vi "FPGA Main v0.vi"() -> ()   [LabVIEW 2017]
uses:
  <vilib>/rvi/Emulation/niFpgaGetClockAttributes.vi
  <vilib>/rvi/Emulation/niFpgaSctlEmulationGetInTimedLoop.vi
  <vilib>/rvi/Emulation/niFpgaEmulationReportErrorSimple.vi
  <vilib>/rvi/eio/common/nirviEmuTemplateMethod_errors.vi
  <vilib>/rvi/Emulation/niFpgaCriticalErrorInLSC.vi
  <vilib>/eio/EIONode/EIONode.xnode
  <vilib>/rvi/FXPMathLib/FxpSub/XNode/nifxpmath_Sub.xnode
  <vilib>/rvi/FXPMathLib/sim/FxpSim.dll
panel:
  in  "DO 1":T1
  out "DI 2":T2
  out "DI 1":T3
  in  "Loop Time (ms)":u32=1 caption="Count(mSec)"
  in  "Stop Button":bool
  out "AI3":fxp<+/-,27,6> format="%.23g"
  out "AI2":fxp<+/-,27,6> format="%.23g"
  out "AI1":fxp<+/-,27,6> format="%.23g"
  out "AI0":fxp<+/-,27,6> format="%.23g"
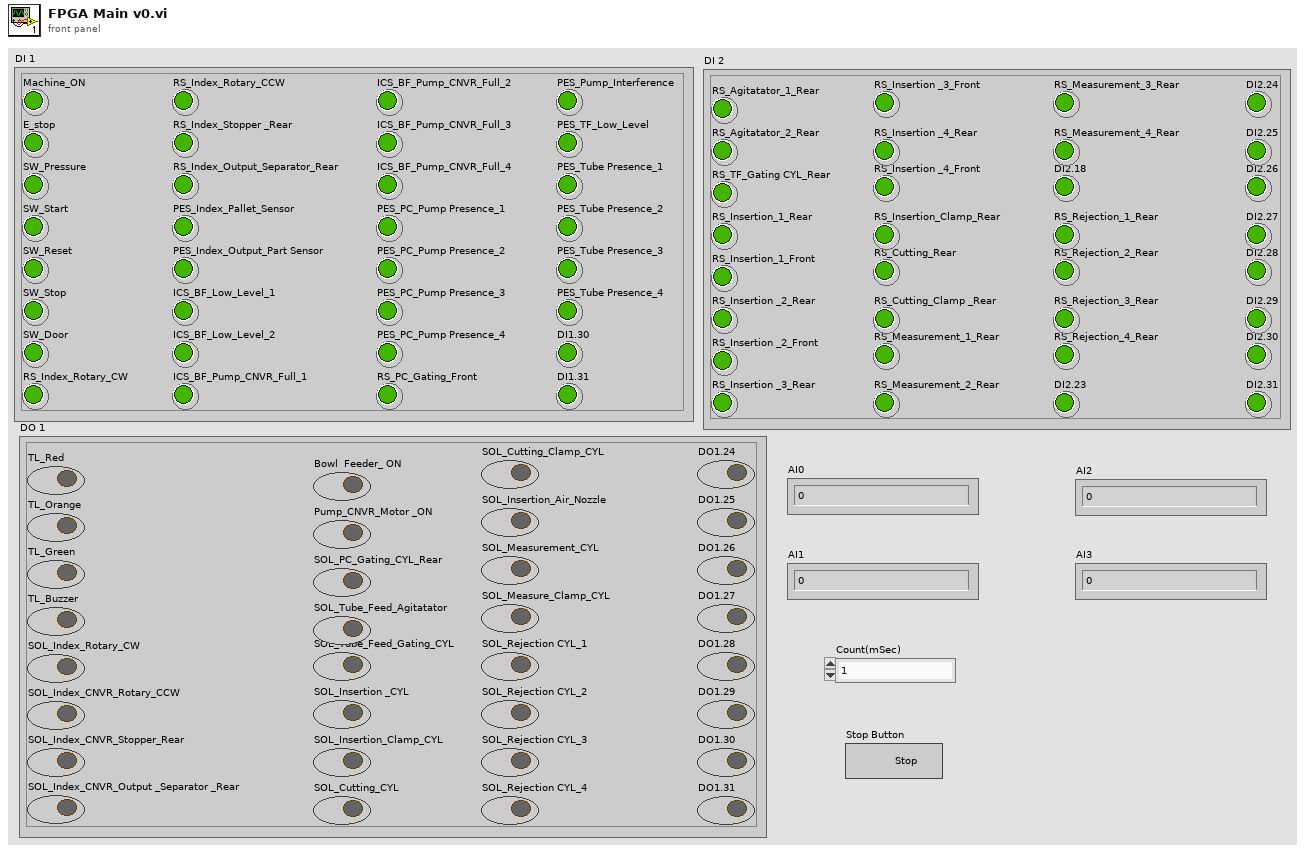
[diagram p1: front panel]
types:
  T1 = cluster{"TL_Red":bool, "TL_Orange":bool, "TL_Green":bool, "TL_Buzzer":bool, "SOL_Index_Rotary_CW":bool, "SOL_Index_CNVR_Rotary_CCW":bool, "SOL_Index_CNVR_Stopper_Rear":bool, "SOL_Index_CNVR_Output _Separator _Rear":bool, "Bowl  Feeder_ ON":bool, "Pump_CNVR_Motor _ON":bool, "SOL_PC_Gating_CYL_Rear":bool, "SOL_Tube_Feed_Agitatator":bool, "SOL_Tube_Feed_Gating_CYL":bool, "SOL_Insertion _CYL":bool, "SOL_Insertion_Clamp_CYL":bool, "SOL_Cutting_CYL":bool, "SOL_Cutting_Clamp_CYL":bool, "SOL_Insertion_Air_Nozzle":bool, "SOL_Measurement_CYL":bool, "SOL_Measure_Clamp_CYL":bool, "SOL_Rejection CYL_1":bool, "SOL_Rejection CYL_2":bool, "SOL_Rejection CYL_3":bool, "SOL_Rejection CYL_4":bool, "DO1.24":bool, "DO1.25":bool, "DO1.26":bool, "DO1.27":bool, "DO1.28":bool, "DO1.29":bool, "DO1.30":bool, "DO1.31":bool}
  T2 = cluster{"RS_Agitatator_1_Rear ":bool, "RS_Agitatator_2_Rear ":bool, "RS_TF_Gating CYL_Rear":bool, "RS_Insertion_1_Rear":bool, "RS_Insertion_1_Front":bool, "RS_Insertion _2_Rear":bool, "RS_Insertion _2_Front":bool, "RS_Insertion _3_Rear":bool, "RS_Insertion _3_Front":bool, "RS_Insertion _4_Rear":bool, "RS_Insertion _4_Front":bool, "RS_Insertion_Clamp_Rear":bool, "RS_Cutting_Rear":bool, "RS_Cutting_Clamp _Rear":bool, "RS_Measurement_1_Rear":bool, "RS_Measurement_2_Rear":bool, "RS_Measurement_3_Rear":bool, "RS_Measurement_4_Rear":bool, "DI2.18":bool, "RS_Rejection_1_Rear":bool, "RS_Rejection_2_Rear":bool, "RS_Rejection_3_Rear":bool, "RS_Rejection_4_Rear":bool, "DI2.23":bool, "DI2.24":bool, "DI2.25":bool, "DI2.26":bool, "DI2.27":bool, "DI2.28":bool, "DI2.29":bool, "DI2.30":bool, "DI2.31":bool}
  T3 = cluster{"Machine_ON":bool, "E_stop ":bool, "SW_Pressure":bool, "SW_Start ":bool, "SW_Reset":bool, "SW_Stop":bool, "SW_Door":bool, "RS_Index_Rotary_CW":bool, "RS_Index_Rotary_CCW":bool, "RS_Index_Stopper _Rear":bool, "RS_Index_Output_Separator_Rear":bool, "PES_Index_Pallet_Sensor":bool, "PES_Index_Output_Part Sensor":bool, "ICS_BF_Low_Level_1":bool, "ICS_BF_Low_Level_2":bool, "ICS_BF_Pump_CNVR_Full_1":bool, "ICS_BF_Pump_CNVR_Full_2":bool, "ICS_BF_Pump_CNVR_Full_3":bool, "ICS_BF_Pump_CNVR_Full_4":bool, "PES_PC_Pump Presence_1":bool, "PES_PC_Pump Presence_2":bool, "PES_PC_Pump Presence_3":bool, "PES_PC_Pump Presence_4":bool, "RS_PC_Gating_Front":bool, "PES_Pump_Interference":bool, "PES_TF_Low_Level":bool, "PES_Tube Presence_1":bool, "PES_Tube Presence_2":bool, "PES_Tube Presence_3":bool, "PES_Tube Presence_4":bool, "DI1.30":bool, "DI1.31":bool}
  T4 = cluster{"Boolean array[0]":bool, "Boolean array[1]":bool, "Boolean array[2]":bool, "Boolean array[3]":bool, "Boolean array[4]":bool, "Boolean array[5]":bool, "Boolean array[6]":bool, "Boolean array[7]":bool, "Boolean array[8]":bool, "Boolean array[9]":bool, "Boolean array[10]":bool, "Boolean array[11]":bool, "Boolean array[12]":bool, "Boolean array[13]":bool, "Boolean array[14]":bool, "Boolean array[15]":bool, "Boolean array[16]":bool, "Boolean array[17]":bool, "Boolean array[18]":bool, "Boolean array[19]":bool, "Boolean array[20]":bool, "Boolean array[21]":bool, "Boolean array[22]":bool, "Boolean array[23]":bool, "Boolean array[24]":bool, "Boolean array[25]":bool, "Boolean array[26]":bool, "Boolean array[27]":bool, "Boolean array[28]":bool, "Boolean array[29]":bool, "Boolean array[30]":bool, "Boolean array[31]":bool}
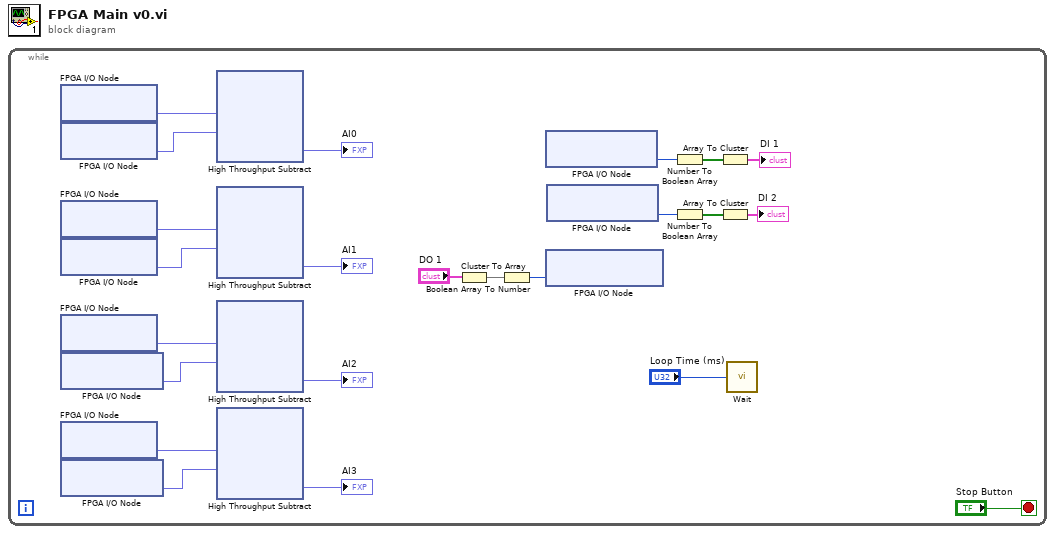
[diagram p0: block diagram]
diagram:
  n1 = while {
    stop <- "Stop Button" stop-if-true
    n2 = xnode "FPGA I/O Node"() -> ("Mod1/AI0"=w23:fxp<+/-,26,5>)  [unwired: 1 in, 1 out]
    n3 = xnode "FPGA I/O Node"() -> ("Mod1/AI8"=w22:fxp<+/-,26,5>)  [unwired: 1 in, 1 out]
    n4 = xnode "FPGA I/O Node"() -> ("Mod1/AI1"=w19:fxp<+/-,26,5>)  [unwired: 1 in, 1 out]
    n5 = xnode "FPGA I/O Node"() -> ("Mod1/AI9"=w18:fxp<+/-,26,5>)  [unwired: 1 in, 1 out]
    n6 = xnode "FPGA I/O Node"() -> ("Mod1/AI2"=w16:fxp<+/-,26,5>)  [unwired: 1 in, 1 out]
    n7 = xnode "FPGA I/O Node"() -> ("Mod1/AI10"=w15:fxp<+/-,26,5>)  [unwired: 1 in, 1 out]
    n8 = xnode "FPGA I/O Node"() -> ("Mod1/AI3"=w13:fxp<+/-,26,5>)  [unwired: 1 in, 1 out]
    n9 = xnode "FPGA I/O Node"() -> ("Mod1/AI11"=w12:fxp<+/-,26,5>)  [unwired: 1 in, 1 out]
    n10 = xnode "High Throughput Subtract"("x"=w23, "y"=w22) -> ("x-y"=→"AI0":fxp<+/-,27,6>)
    n11 = xnode "High Throughput Subtract"("x"=w19, "y"=w18) -> ("x-y"=→"AI1":fxp<+/-,27,6>)
    n12 = xnode "High Throughput Subtract"("x"=w16, "y"=w15) -> ("x-y"=→"AI2":fxp<+/-,27,6>)
    n13 = xnode "High Throughput Subtract"("x"=w13, "y"=w12) -> ("x-y"=→"AI3":fxp<+/-,27,6>)
    n14 = Cluster To Array(cluster="DO 1") -> (array=w3:bool[])
    n15 = Boolean Array To Number(Boolean array=w3) -> (number=w8:u32)
    n16 = xnode "FPGA I/O Node"() -> ("Mod2/DI31:0"=w10:u32)  [unwired: 1 in, 1 out]
    n17 = xnode "FPGA I/O Node"("Mod4/DO31:0"=w8) -> ()  [unwired: 1 in, 1 out]
    n18 = xnode "FPGA I/O Node"() -> ("Mod3/DI31:0"=w9:u32)  [unwired: 1 in, 1 out]
    n19 = Number To Boolean Array(number=w10) -> (Boolean array=w6:bool[])
    n20 = Number To Boolean Array(number=w9) -> (Boolean array=w2:bool[])
    n21 = Array To Cluster(array=w6) -> (cluster=→"DI 1":T4)
    n22 = Array To Cluster(array=w2) -> (cluster=→"DI 2":T4)
    n23 = call "Wait"("Count(mSec)"="Loop Time (ms)") -> ()  [unwired: 1 out]
  }
